vi "Multi-Device Rx Streaming Time (Host).vi"() -> ()   [LabVIEW 2015]
doc: "This template is for the Simple NI-USRP Streaming design, a design that shows the basics of streaming data to and from an NI USRP-294x/295x device. Refer to the block diagram for more information about how to use this template."
uses:
  <vilib>/Utility/error.llb/DialogType.ctl
  <vilib>/userdefined/Silver/nirio_resource_slv.ctl
  SubVIs/Start Trigger.ctl
panel:
  in  "config tab":enum32{"Rx Configuration"}(tab)
  in  "rx config":T2={"rf enable 0"=TRUE, "rf config 0"={"antenna"="RX2", "frequency"=2000000000.0, "lo frequency"=-1.0, "level"=0.0}, "rf enable 1"=TRUE, "rf config 1"={"antenna"="RX2", "frequency"=2000000000.0, "lo frequency"=-1.0, "level"=0.0}, "transfer mode"=enum."Finite", "sample rate"=10000000.0, "number of samples"=8192, "start trigger"=enum."Future Time Event"} {"sample rate" format="%#.3pS/s"; "rf config 1"."level" format="%#_gdBm"; "rf config 1"."lo frequency" format="%#.3pHz"; "rf config 1"."frequency" format="%#.3pHz"; "rf config 0"."level" format="%#_gdBm"; "rf config 0"."lo frequency" format="%#.3pHz"; "rf config 0"."frequency" format="%#.3pHz"}
  out "acquiring":bool caption="Acquiring"
  in  "USRP RIO devices":T3[](array[typedef])=["RIO0", "RIO1"] caption="USRP RIO Devices"
  in  "reference frequency source":string(combo)="REF IN" caption="Reference Frequency Source"
  in  "indicator tab":T4(tab)
  out "power spectrum":cluster{"f0":dbl, "df":dbl, "magnitude":dbl[]}[](graph) caption="Power Spectrum"
  out "power level":dbl[][](graph) caption="Power Level"
  out "iq data":waveform(dbl)[](graph) caption="I & Q Data"
  out "rx.coerced config":T5(array[cluster]) caption="Rx" {"coerced sample rates" format="%#.3pS/s"; "coerced levels" format="%#.3gdBm"; "coerced lo frequencies" format="%#.3pHz"; "coerced frequencies" format="%#.3pHz"}
  in  "rx.stop":bool
  # "This template is for the Simple NI-USRP Streaming design, a design that shows the basics of streaming data on an NI 294x/295x device. See the block diagram for more information on how to use this template."
  # "Multi-Device Rx Streaming with Time"
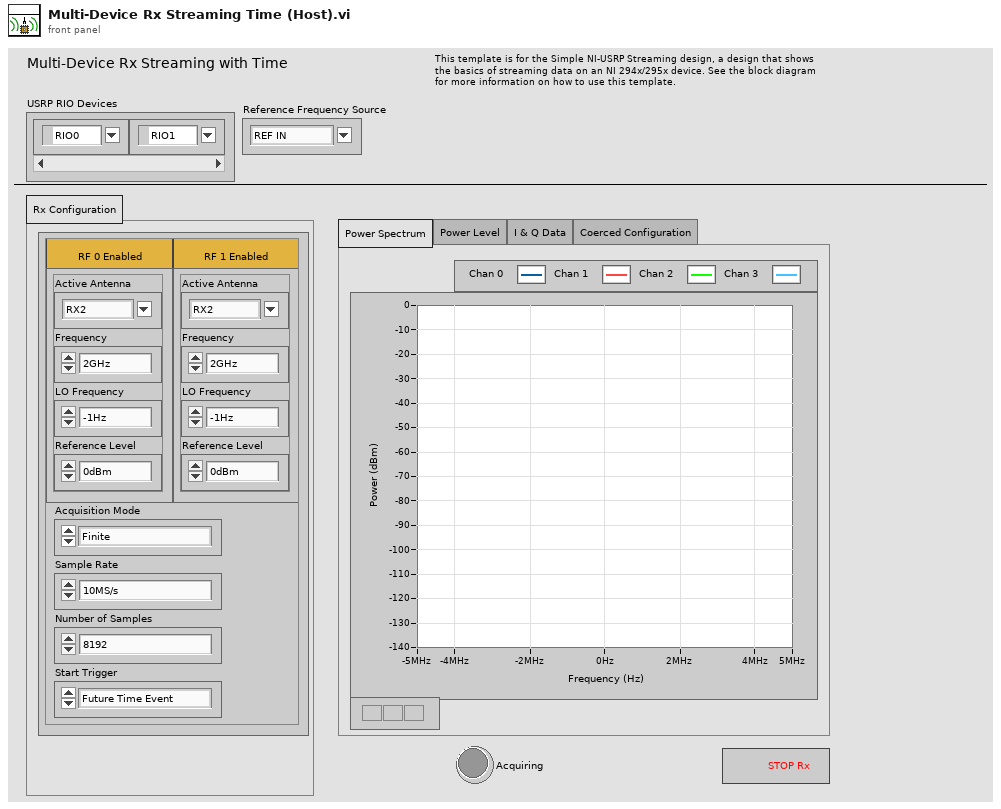
[diagram p1: front panel]
types:
  T1 = typedef "Start Trigger.ctl" = enum8{"Software", "Digital Edge", "Rx Start Trigger", "Tx Start Trigger", "Immediate", "Future Time Event"}
  T2 = cluster{"rf enable 0":bool, "rf config 0":cluster{"antenna":string, "frequency":dbl, "lo frequency":dbl, "level":dbl}, "rf enable 1":bool, "rf config 1":cluster{"antenna":string, "frequency":dbl, "lo frequency":dbl, "level":dbl}, "transfer mode":enum16{"Finite", "Continuous"}, "sample rate":dbl, "number of samples":u32, "start trigger":T1}
  T3 = typedef "nirio_resource_slv.ctl" = tag
  T4 = enum32{"Power Spectrum", "Power Level", "I & Q Data", "Coerced Configuration"}
  T5 = cluster{"coerced frequencies":dbl[], "coerced lo frequencies":dbl[], "coerced levels":dbl[], "coerced sample rates":dbl[]}[]
  T6 = typedef "DialogType.ctl" = u16
  T7 = cluster{"rx config":cluster{"rf enable 0":bool, "rf config 0":cluster{"antenna":string, "frequency":dbl, "lo frequency":dbl, "level":dbl}, "rf enable 1":bool, "rf config 1":cluster{"antenna":string, "frequency":dbl, "lo frequency":dbl, "level":dbl}, "transfer mode":enum16{"Finite", "Continuous"}, "sample rate":dbl, "number of samples":u32, "start trigger":T1}, "reference frequency source":string, "rx.enabled channels":string[], "vertical range":dbl[], "rx.coerced configurations":cluster{"coerced frequencies":dbl[], "coerced lo frequencies":dbl[], "coerced levels":dbl[], "coerced sample rates":dbl[]}}
  T8 = typedef "niUsrpRio Config v1 Host.lvlib/niUsrpRio Session.ctl" = cluster{"FPGA Interface":refnum<k20>, "RIO Interface Number":u32, "Data Clock Rate":u32, "FPGA Data Clock Rate":u32, "Global Settings Register Bus":T9, "Radio 0 Settings Register Bus":T9, "Radio 1 Settings Register Bus":T9, "Radio Settings Bus Semaphore":T10, "DB Queues":T11[], "Characterization Data Valid?":bool, "EEPROM Header":T12, "Device Data Header":T13, "EEPROM Characterization Header":T14, "Characterization Data":T15[], "FPGA Current Version":u32, "FPGA Oldest Compatible Version":u32, "Fixed Logic Current Version":u32, "Fixed Logic Oldest Compatible Version":u32, "FPGA Radio Settings Bus Current Version":u32, "FPGA Radio Settings Bus Oldest Compatible Version":u32, "FPGA Board Config Current Version":u32, "FPGA Board Config Oldest Compatible Version":u32, "Daughterboard Clock Rate":u32}
  T9 = typedef "niInstr Register Bus v0 Host.lvlib/Register Bus Session.ctl" = refnum<queue>
  T10 = typedef "Semaphore RefNum" = refnum<k1>
  T11 = typedef "niUsrpRio Config v1 Host.lvlib/DB Queue Reference.ctl" = refnum<queue>
  T12 = typedef "niUsrpRio Config v1 Host.lvlib/EEPROM Header.ctl" = cluster{"Checksum":u32, "Product Code":u16, "Hardware Current Version":u16, "Hardware Oldest Compatible Version":u16, "EEPROM Map Current Version":u16, "EEPROM Map Oldest Compatible Version":u16, "User Password":string, "Pointer to Factory Header":u32, "Pointer to User Header":u32, "Recommended Interval":u16, "Number of Reserved Bytes":i32, "Number of Daughterboards":u8, "Daughterboard IDs":u16[], "Daughterboard Serial Numbers":string[]}
  T13 = typedef "niUsrpRio Config v1 Host.lvlib/EEPROM Device Data Header.ctl" = cluster{"Checksum":u32, "Number of Channels":u8, "Number of Gain Settings":u16[], "Pointer to Characterization Data":u32[], "Number of Reserved Bytes":i32, "Number of Frequencies":u16[]}
  T14 = typedef "niUsrpRio Config v1 Host.lvlib/EEPROM Characterization Header.ctl" = cluster{"Checksum":u32, "Date":timestamp, "Temperature":sgl, "Misc. Info":string, "Pointer to Device Data Header":u32, "Number of Reserved Bytes":i32}
  T15 = typedef "niUsrpRio Config v1 Host.lvlib/Characterization Data.ctl" = cluster{"Gains[dB]":dbl[], "Frequencies [Hz]":dbl[], "IQ Imbalance Table":T16[], "Measured Gains[dB]":dbl[][]}
  T16 = typedef "niUsrpRio Config v1 Host.lvlib/IQ Imbalance.ctl" = cluster{"Gain Imbalance [linear]":dbl, "Phase Imbalance [radians]":dbl, "Offset":cdb}
  T17 = cluster{"coerced frequencies":dbl[], "coerced lo frequencies":dbl[], "coerced levels":dbl[], "coerced sample rates":dbl[]}
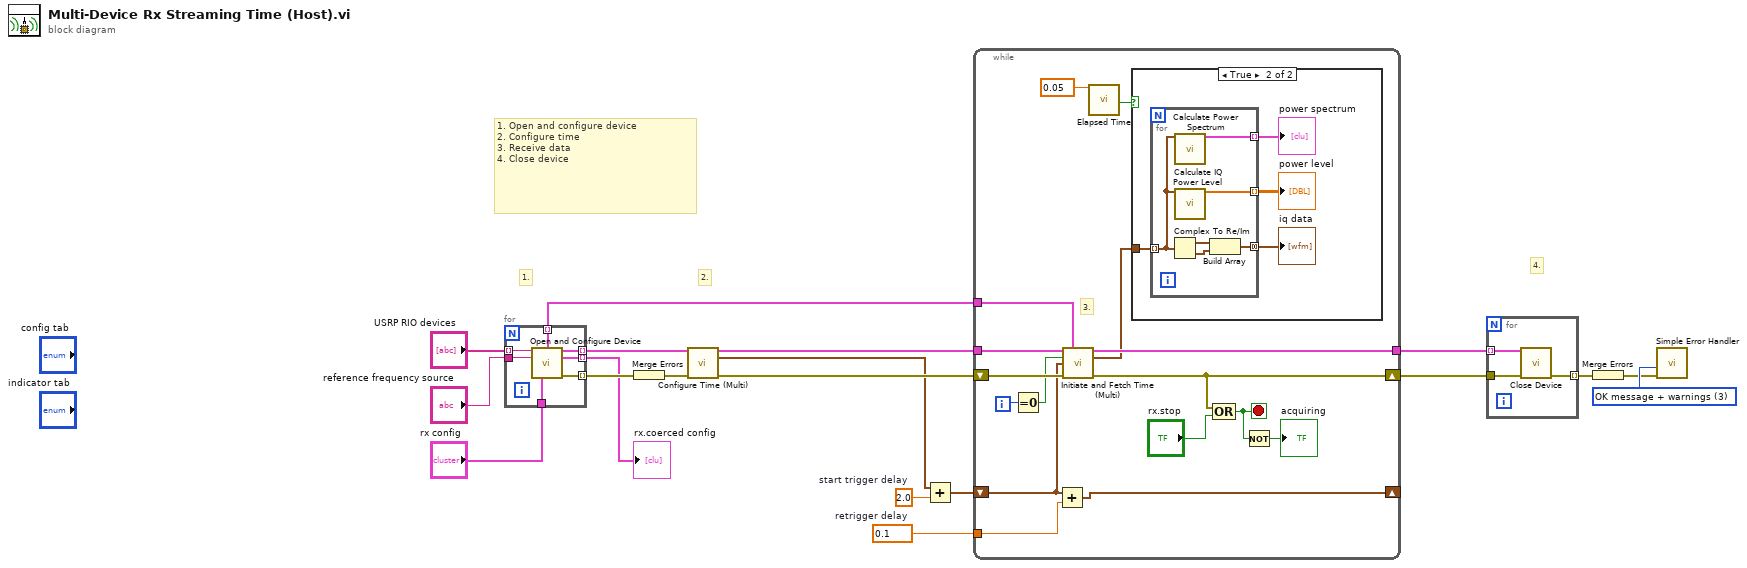
[diagram p0: block diagram]
diagram:
  w3 = 2.0  # start trigger delay
  w2 = 0.1  # retrigger delay
  w16 = T6 3 items=["no dialog", "OK message", "continue or stop message", "OK message + warnings", "continue/stop + warnings"] ("type of dialog (OK msg:1)")
  # "4."
  # "2."
  # "1. Open and configure device\n2. Configure time\n3. Receive data\n4. Close device"
  # "1."
  n1 = for {
    tunnel: [w26] -> w17 mode=indexing
    tunnel: [w25] -> w14 mode=indexing
    tunnel: "rx config" -> [w24]
    tunnel: "reference frequency source" -> [w23]
    tunnel: [w22] -> w7 mode=indexing
    tunnel: [w21] -> w11 mode=indexing
    tunnel: "USRP RIO devices" -> [w20] mode=indexing
    n2 = call "Open and Configure Device.vi"("USRP RIO Device"=w20, "reference frequency source"=w23, "rx config"=w24) -> ("rx channels"=w25:T7, "niUsrpRio Session (out)"=w21:T8, "rx.coerced configurations"=w22:T17, "error out"=w26:errorcluster)  [unwired: 6 in, 3 out]
  }
  "rx.coerced config" <- w7
  n3 = Merge Errors(w17) -> (w4:errorcluster)
  n4 = call "Configure Time (Multi).vi"("niUsrpRio Sessions"=w11, "error in"=w4) -> ("niUsrpRio Sessions (out)"=w10:T8[], "time"=w18:timestamp, "error out"=w19:errorcluster)  [unwired: 11 in]
  n5 = Add(x=w18, y=w3) -> (x+y=w1:timestamp)
  n6 = while {
    tunnel: w10 -> [w40]
    tunnel: [w37] -> w5
    tunnel: w14 -> [w34]
    shift-right: [w38] -> w6
    shift-left: w19 -> [w41]
    tunnel: w2 -> [w28]
    shift-right: [w27] -> _
    shift-left: w1 -> [w29]
    i -> [w39]
    stop <- w35 stop-if-true
    # "3."
    # "Acquire and Fetch a waveform"
    n7 = Equal To 0?(x=w39) -> (x = 0?=w30:bool)
    n8 = Add(x=w29, y=w28) -> (x+y=w27:timestamp)
    n9 = call "Initiate and Fetch Time (Multi).vi"("niUsrpRio Sessions"=w40, "rx channels"=w34, "first iteration"=w30, "start trigger time"=w29, "error in"=w41) -> ("niUsrpRio Sessions (out)"=w37:T8[], "complex baseband data"=w31:waveform(cdb)[], "error out"=w38:errorcluster)  [unwired: 8 in]
    n10 = call "Elapsed Time"("Time Target (s)"=0.05 ("retrigger delay")) -> ("Time has Elapsed"=w32:bool)  [unwired: 11 in, 7 out]
    n11 = case shown="True" w32 {
      tunnel: w31 -> [_ w46]
      frame False {
      }
      frame True {
        n12 = for {
          tunnel: [w50] -> w45 mode=concatenating
          tunnel: [w49] -> w44 mode=indexing
          tunnel: [w48] -> w43 mode=indexing
          tunnel: w46 -> [w47] mode=indexing
          n13 = Complex To Re/Im(x + iy=w47) -> (x=w52:waveform(dbl), y=w51:waveform(dbl))
          n14 = call "Calculate Power Spectrum.vi"("waveform"=w47) -> ("power spectrum (dBm)"=w48:cluster{"f0":dbl, "df":dbl, "magnitude":dbl[]})  [unwired: 14 in]
          n15 = call "Calculate IQ Power Level.vi"("iq data"=w47) -> ("power level (dBm)"=w49:dbl[])  [unwired: 14 in]
          n16 = Build Array(w52, w51) -> (w50:waveform(dbl)[])
        }
        "power level" <- w44
        "power spectrum" <- w43
        "iq data" <- w45
      }
    }
    n17 = Compound Arithmetic op=OR(w38, "rx.stop") -> (w35:bool)
    n18 = Not(x=w35) -> (.not. x?=→"acquiring":bool)
  }
  n19 = for {
    tunnel: w5 -> [w53] mode=indexing
    tunnel: w6 -> [w54]
    tunnel: [w55] -> w15 mode=indexing
    n20 = call "Close Device.vi"("niUsrpRio Session"=w53, "error in"=w54) -> ("error out"=w55:errorcluster)  [unwired: 13 in]
  }
  n21 = Merge Errors(w15) -> (w8:errorcluster)
  n22 = call <vilib>:"Simple Error Handler.vi"("type of dialog (OK msg:1)"=w16, "error in (no error)"=w8) -> ()  [unwired: 3 in, 5 out]
